vi "Validate Connection.vi"(0 "connection ID in":refnum<k5>, 11 "Error In":errorcluster) -> (4 "connection ID out":refnum<k5>, 8 "Valid?":bool, 15 "Error Out":errorcluster)   [LabVIEW 2014, in "hse-db.lvlib" / "MySQL (TCP).lvlib"]
uses:
  MySQL (TCP).lvlib
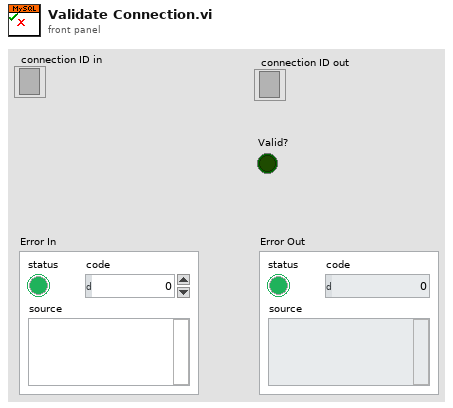
[diagram p1: front panel]
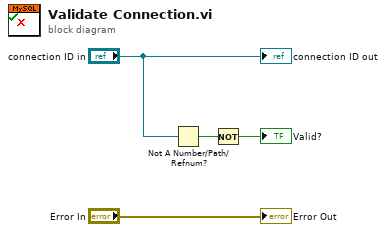
[diagram p0: block diagram]
diagram:
  n1 = Not A Number/Path/Refnum?(number/path/refnum="connection ID in") -> (NaN/Path/Refnum?=w2:bool)
  n2 = Not(x=w2) -> (.not. x?=→"Valid?":bool)
  "connection ID out" <- "connection ID in"
  "Error Out" <- "Error In"
